vi "Ignore-error-multiple.vi"(8 "error in (no error)":errorcluster, 10 "Errors to ignore (1)":i32[](array[numeric])) -> (0 "error out":errorcluster)   [LabVIEW 2013, in "CameraVision.lvlib" / "CV-Client.lvclass"]
uses:
  CV-Client.lvclass
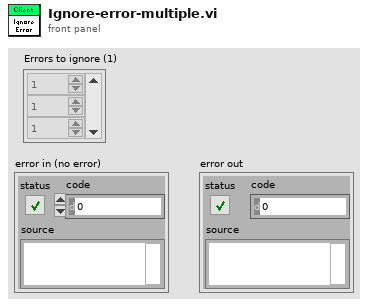
[diagram p1: front panel]
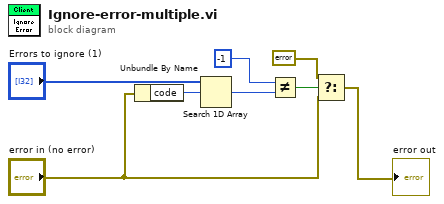
[diagram p0: block diagram]
diagram:
  n1 = Unbundle By Name("error in (no error)") -> ("code"=w3:i32)
  n2 = Search 1D Array(1D array="Errors to ignore (1)", element=w3) -> (index of element=w2:i32)  [unwired: 1 in]
  n3 = Not Equal?(x=-1, y=w2) -> (x != y?=w5:bool)
  n4 = Select(t=errorcluster {"status"=FALSE, "code"=0, "source"=""} ("error constant"), s=w5, f="error in (no error)") -> (s? t:f=→"error out":errorcluster)
